vi "Module (Top Level).vi"(8 "error in":errorcluster) -> (0 "error out":errorcluster)   [LabVIEW 2017, in "WinHost.lvlib"]
uses:
  WinHost.lvlib
  User Events/TypeDefs/Shutdown UE FGV Command.ctl
  Global TypeDefs/Registered Modules.ctl
  Public TypeDefs/Messages.ctl
  Public TypeDefs/Module Events.ctl
  <vilib>/NI/STM/SubVIs/MetaDataElement.ctl
  Private TypeDefs/STM Queue Element.ctl
  <vilib>/NI/STM/TCP/TCP Read Options.ctl
  <vilib>/NI/STM/TCP/Write Meta Data (TCP Ref).vi
  <vilib>/NI/STM/TCP/Write Meta Data (TCP Clst).vi
  <vilib>/NI/STM/TCP/Write Message (TCP).vi
  <vilib>/NI/STM/TCP/Read Message (TCP).vi
  Error Handler/Error Handler.lvlib
  Logger/Logger.lvlib
  Controller/Controller.lvlib
  <vilib>/NI/STM/NI STM.lvlib
  mypam/myPAM.lvlib
  Game/Game.lvlib
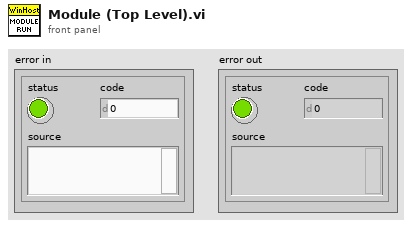
[diagram p1: front panel]
types:
  T1 = typedef "Registered Modules.ctl" = enum16{"Controller", "DAQ", "Error Handler", "Game", "myPAM", "WinHost", "Logger"}
  T2 = typedef "Shutdown UE FGV Command.ctl" = enum16{"create", "get", "destroy"}
  T3 = typedef "Controller.lvlib/Module Reference.ctl" = cluster{"calling module":T1, "module queues":T4, "module notifiers":T5}
  T4 = typedef "Controller.lvlib/Module Queues.ctl" = cluster{"message queue":refnum<queue>}
  T5 = typedef "Controller.lvlib/Module Notifiers.ctl" = cluster{"dummy notifier":refnum<notifier>}
  T6 = typedef "Logger.lvlib/Module Reference.ctl" = cluster{"calling module":T1, "module queues":T7, "module notifiers":T8}
  T7 = typedef "Logger.lvlib/Module Queues.ctl" = cluster{"message queue":refnum<queue>}
  T8 = typedef "Logger.lvlib/Module Notifiers.ctl" = cluster{"dummy notifier":refnum<notifier>}
  T9 = typedef "WinHost.lvlib/Module Reference.ctl" = cluster{"calling module":T1, "module queues":T10, "module notifiers":T11}
  T10 = typedef "WinHost.lvlib/Module Queues.ctl" = cluster{"message queue":refnum<queue>, "STM queue":refnum<queue>}
  T11 = typedef "WinHost.lvlib/Module Notifiers.ctl" = cluster{"dummy notifier":refnum<notifier>}
  T12 = typedef "Error Handler.lvlib/Module Reference.ctl" = cluster{"calling module":T1, "module queues":T13, "module notifiers":T14}
  T13 = typedef "Error Handler.lvlib/Module Queues.ctl" = cluster{"message queue":refnum<queue>}
  T14 = typedef "Error Handler.lvlib/Module Notifiers.ctl" = cluster{"dummy notifier":refnum<notifier>}
  T15 = typedef "WinHost.lvlib/Module Events.ctl" = enum16{"host connected", "enable assistance", "disable assistance", "host disconnected"}
  T16 = typedef "WinHost.lvlib/STM Queue Element.ctl" = cluster{"name":string, "data":string, "stop":bool}
  T17 = typedef "NI STM.lvlib/TCP Read Options.ctl" = cluster{"ignore timeout error":bool, "timeout ms (1000)":i32}
  T18 = typedef "WinHost.lvlib/Messages.ctl" = enum16{"shutdown", "wait for host", "communicate"}
  T19 = typedef "NI STM.lvlib/MetaDataElement.ctl" = string
  T20 = typedef "NI STM.lvlib/TCP Connection Info.ctl" = cluster{"connection ID":refnum<k5>, "meta data":T19[]}
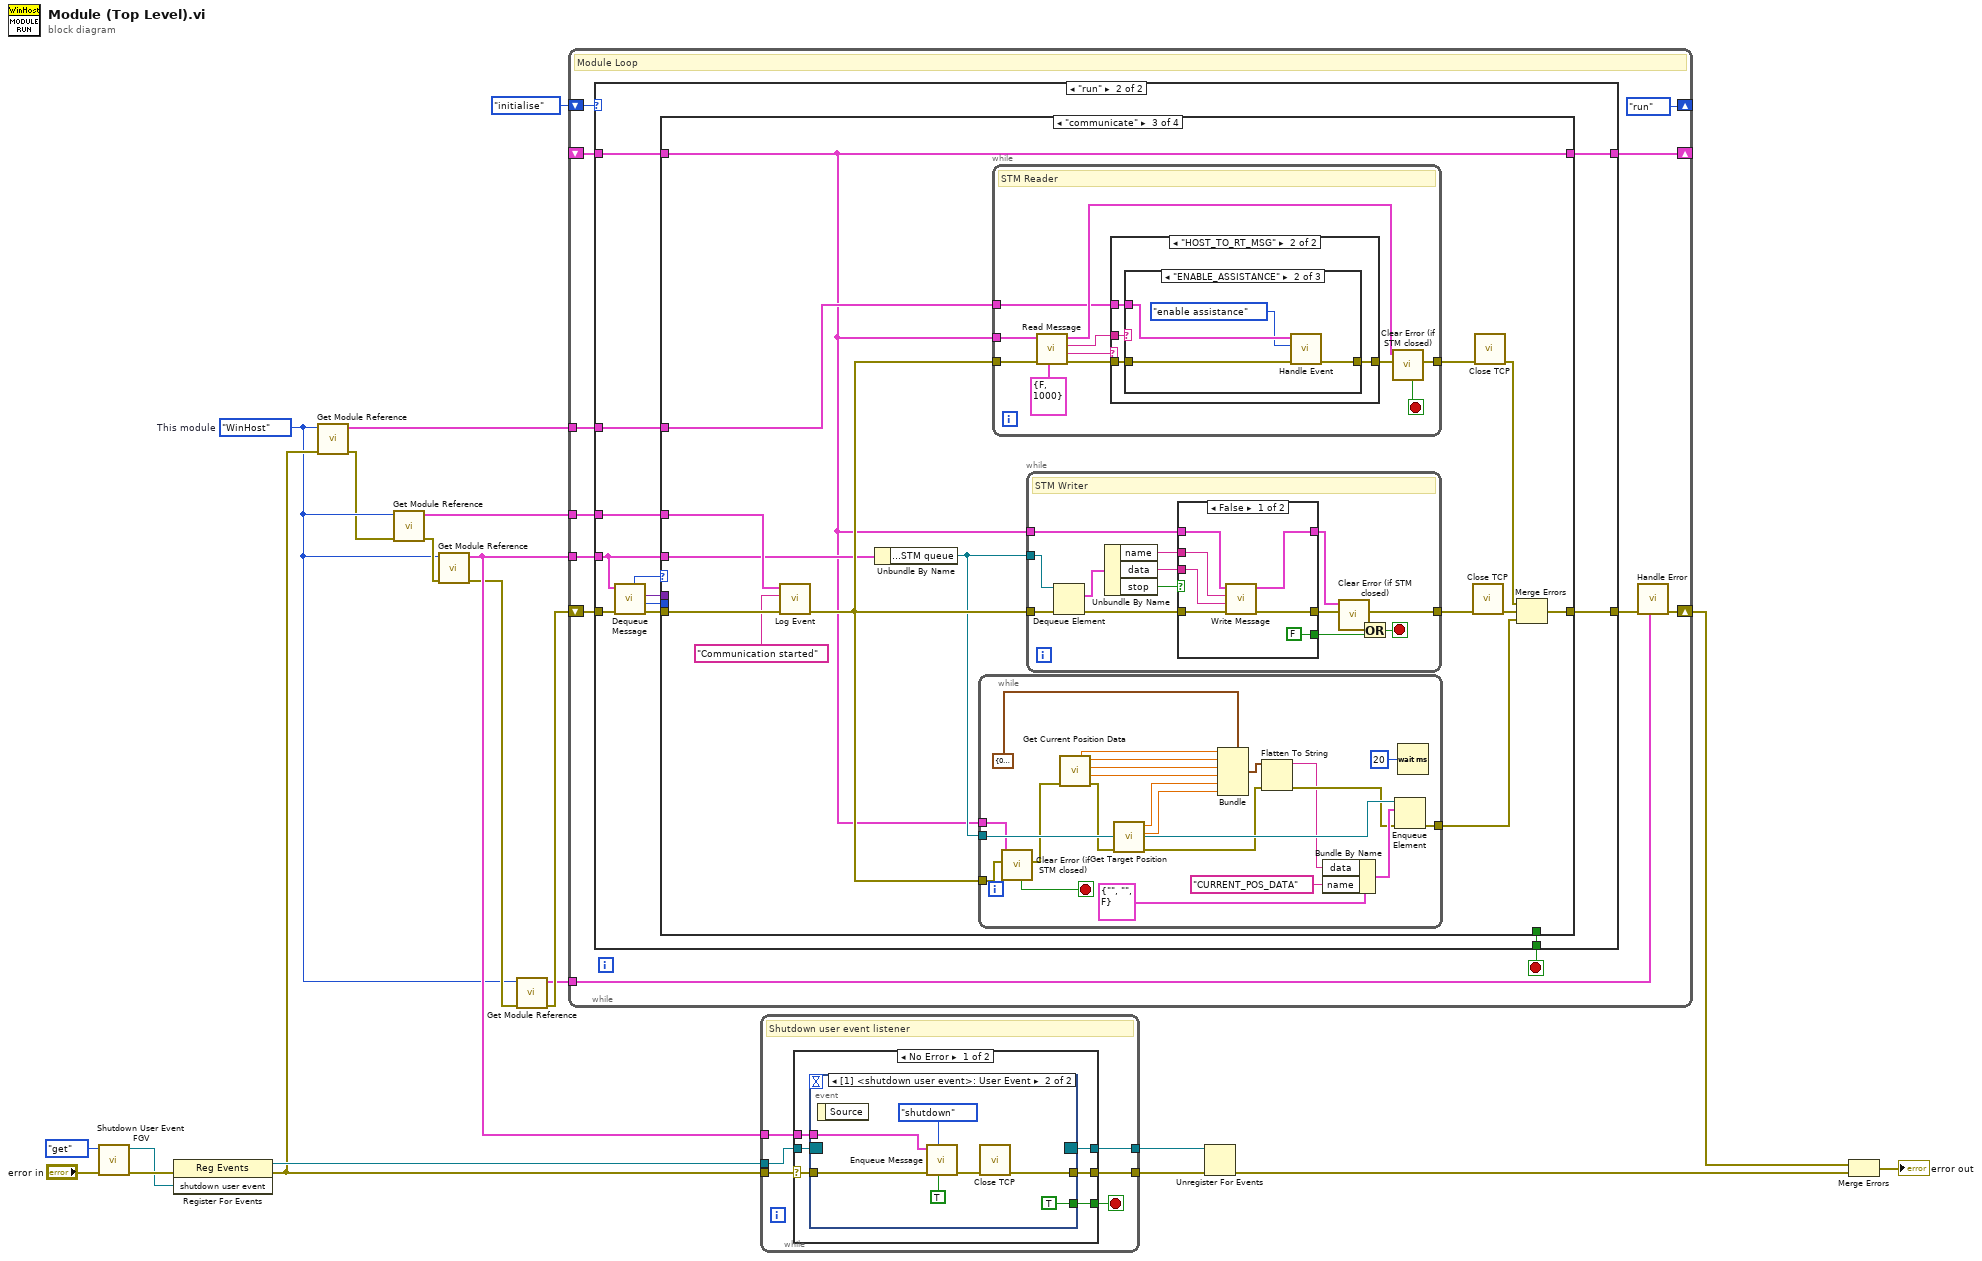
[diagram p0: block diagram]
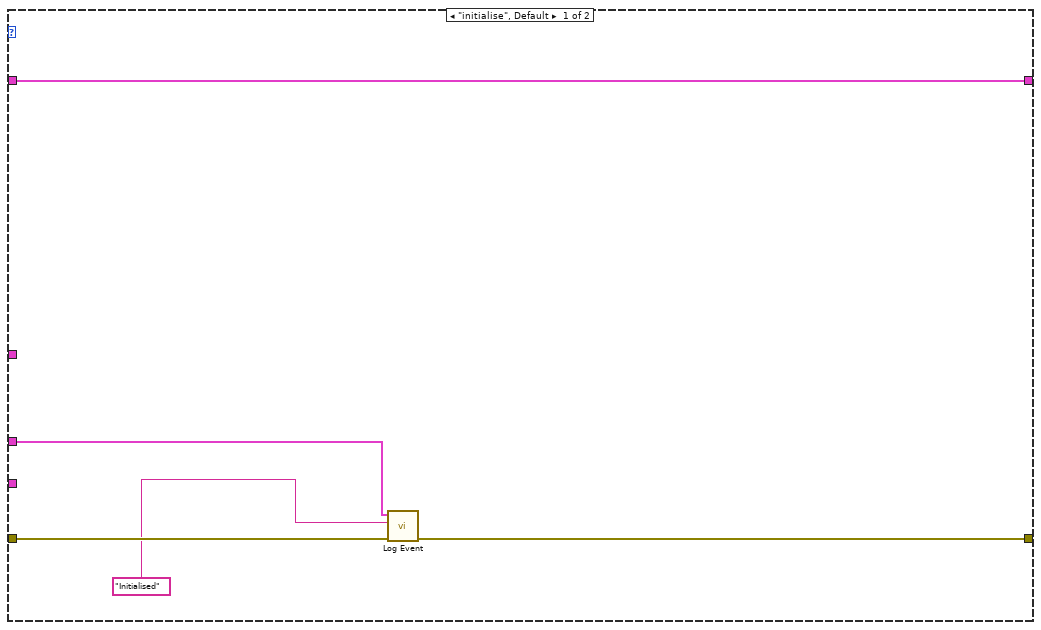
[diagram p2: hidden frame]
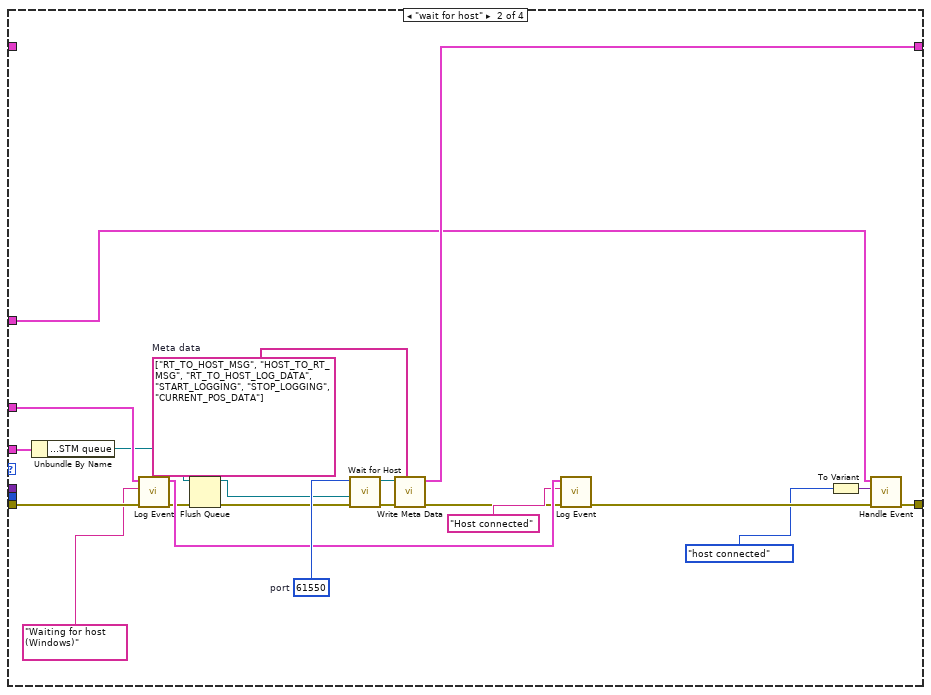
[diagram p4: hidden frame]
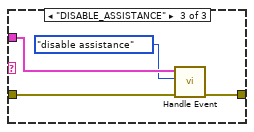
[diagram p7: hidden frame]
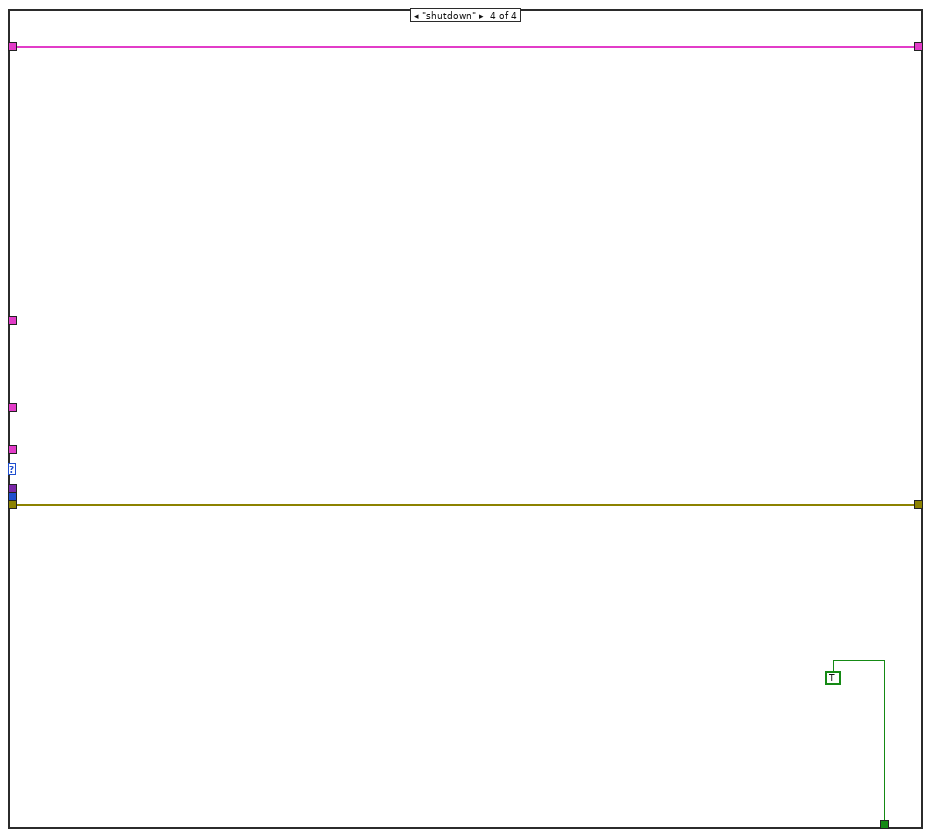
[diagram p9: hidden frame]
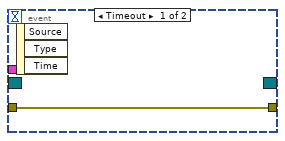
[diagram p10: hidden frame]
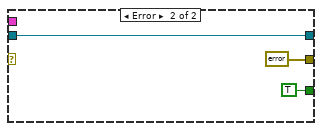
[diagram p11: hidden frame]
diagram:
  w3 = Registered_Modules."WinHost"  # This module
  n1 = call "Shutdown User Event FGV.vi"("error in"="error in", "command"=Shutdown_UE_FGV_Command."get" ("Command")) -> ("error out"=w17:errorcluster, "shutdown user event"=w16:refnum<user-event>)  [unwired: 8 in]
  n2 = register-events(error in=w17, w16) -> (reference out=w20:refnum<event-registration>, error out=w4:errorcluster)  [unwired: 1 in]
  n3 = call "Get Module Reference.vi"("error in"=w4, "calling module"=w3) -> ("error out"=w2:errorcluster, "module reference"=w1:T3)  [unwired: 8 in]
  n4 = call "Get Module Reference.vi"("error in"=w2, "calling module"=w3) -> ("error out"=w9:errorcluster, "module reference"=w11:T6)  [unwired: 8 in]
  n5 = call "Get Module Reference.vi"("error in"=w9, "calling module"=w3) -> ("error out"=w7:errorcluster, "module reference"=w12:T9)  [unwired: 8 in]
  n6 = call "Get Module Reference.vi"("error in"=w7, "calling module"=w3) -> ("error out"=w6:errorcluster, "module reference"=w5:T12)  [unwired: 8 in]
  n7 = while {
    shift-right: [w29] -> w10
    shift-left: w6 -> [w27]
    tunnel: w12 -> [w33]
    tunnel: w11 -> [w32]
    shift-right: [enum16{"initialise", "run"}."run"] -> _
    shift-left: enum16{"initialise", "run"}."initialise" -> [w31]
    tunnel: w5 -> [w25]
    shift-right: [w24] -> _
    shift-left: _ -> [w23]
    tunnel: w1 -> [w22]
    stop <- w26 stop-if-true
    # "Module Loop"
    n8 = case shown="\"run\"" w31 {
      tunnel: [w37 w50] -> w30
      tunnel: w33 -> [_ w40]
      tunnel: w32 -> [w36 w45]
      tunnel: w27 -> [w38 w44]
      tunnel: [_ w43] -> w26
      tunnel: [w34 w42] -> w24
      tunnel: w23 -> [w34 w41]
      tunnel: w22 -> [_ w39]
      frame "initialise", Default {
        n9 = call "Log Event.vi"("error in"=w38, "event"="Initialised", "module reference in"=w36) -> ("error out"=w37:errorcluster)  [unwired: 7 in, 1 out]
      }
      frame "run" {
        n10 = call "Dequeue Message.vi"("error in"=w44, "module reference in"=w40) -> ("error out"=w48:errorcluster, "source"=w46:T1, "data"=w47:variant, "message"=w49:T18)  [unwired: 5 in, 1 out]
        n11 = case shown="\"communicate\"" w49 {
          tunnel: [w52 w66 w84 w161] -> w50
          tunnel: w48 -> [w52 w73 w82 w161]
          tunnel: w47 -> [_ _ _ _]
          tunnel: w46 -> [_ _ _ _]
          tunnel: w45 -> [_ w72 w81 _]
          tunnel: [_ _ _ TRUE] -> w43
          tunnel: [w51 w59 w74 w159] -> w42
          tunnel: w41 -> [w51 _ w74 w159]
          tunnel: w40 -> [_ w58 w75 _]
          tunnel: w39 -> [_ w54 w79 _]
          frame Default {
          }
          frame "wait for host" {
            w63 = T19[] ["RT_TO_HOST_MSG", "HOST_TO_RT_MSG", "RT_TO_HOST_LOG_DATA", "START_LOGGING", "STOP_LOGGING", "CURRENT_POS_DATA"]  # Meta data
            w70 = u16 61550  # port
            n12 = Unbundle By Name(w58) -> ("module queues.STM queue"=w55:refnum<queue>)
            n13 = call "Log Event.vi"("error in"=w73, "event"="Waiting for host (Windows)", "module reference in"=w72) -> ("error out"=w56:errorcluster, "module reference out"=w69:T6)  [unwired: 7 in]
            n14 = Flush Queue(queue=w55, error in (no error)=w56) -> (queue out=w53:refnum<queue>, error out=w57:errorcluster)  [unwired: 1 out]
            n15 = call "Wait for Host.vi"("error in"=w57, "STM queue"=w53, "local tcp port"=w70) -> ("error out"=w62:errorcluster, "connection ID"=w61:refnum<k5>)  [unwired: 7 in]
            n16 = call-poly <vilib>:"Write Meta Data.vi"("meta data"=w63, "error in"=w62, "connection ID"=w61) -> ("error out"=w60:errorcluster, "connection info out"=w59:T20)  [unwired: 2 in, 5 out]
            n17 = call "Log Event.vi"("error in"=w60, "event"="Host connected", "module reference in"=w69) -> ("error out"=w67:errorcluster)  [unwired: 7 in, 1 out]
            n18 = To Variant(anything=Module_Events."host connected" ("module events")) -> (Variant=w65:variant)
            n19 = call "Handle Event.vi"("error in"=w67, "event"=w65, "module reference in"=w54) -> ("error out"=w66:errorcluster)  [unwired: 7 in, 1 out]
          }
          frame "communicate" {
            n20 = call "Log Event.vi"("error in"=w82, "event"="Communication started", "module reference in"=w81) -> ("error out"=w78:errorcluster)  [unwired: 7 in, 1 out]
            n21 = Unbundle By Name(w75) -> ("module queues.STM queue"=w77:refnum<queue>)
            n22 = while {
              tunnel: w78 -> [w96]
              tunnel: w77 -> [w109]
              tunnel: [w107] -> w76
              tunnel: w74 -> [w97]
              stop <- w89 stop-if-true
              n23 = call "Clear Error (if STM closed).vi"("error in"=w96, "stm connection"=w97) -> ("error out"=w95:errorcluster, "stop?"=w89:bool)  [unwired: 8 in]
              n24 = call "Get Current Position Data.vi"("error in"=w95) -> ("link 1 x (mm)"=w106:dbl, "link 1 y (mm)"=w88:dbl, "link 2 x (mm)"=w105:dbl, "link 2 y (mm)"=w104:dbl, "error out"=w94:errorcluster)  [unwired: 10 in]
              n25 = call "Get Target Position.vi"("error in"=w94) -> ("error out"=w93:errorcluster, "target y (mm)"=w90:dbl, "target x (mm)"=w91:dbl)  [unwired: 8 in]
              n26 = Bundle(cluster=cluster{dbl, dbl, dbl, dbl, dbl, dbl} {0.0, 0.0, 0.0, 0.0, 0.0, 0.0}, w106, w88, w105, w104, w91, w90) -> (w101:cluster{dbl, dbl, dbl, dbl, dbl, dbl})
              n27 = Flatten To String(anything=w101, error in (no error)=w93) -> (data string=w99:string, error out=w100:errorcluster)  [unwired: 2 in, 1 out]
              n28 = Bundle By Name(cluster=T16 {"name"="", "data"="", "stop"=FALSE} ("element"), "data"=w99, "name"="CURRENT_POS_DATA") -> (w102:T16)
              n29 = Enqueue Element(queue=w109, element=w102, error in (no error)=w100) -> (error out=w107:errorcluster)  [unwired: 1 in, 2 out]
              n30 = Wait (ms)(milliseconds to wait=u32 20) -> ()  [unwired: 1 out]
            }
            n31 = while {
              tunnel: w74 -> [w120]
              tunnel: w78 -> [w118]
              tunnel: [w113] -> w86
              tunnel: w79 -> [w111]
              stop <- w114 stop-if-true
              # "STM Reader"
              n32 = call-poly <vilib>:"Read Message.vi"("options"=T17 {"ignore timeout error"=FALSE, "timeout ms (1000)"=1000}, "error in"=w118, "connection info in"=w120) -> ("error out"=w116:errorcluster, "name"=w110:T19, "data string"=w117:string, "connection info out"=w112:T20)  [unwired: 3 in, 2 out]
              n33 = case shown="\"HOST_TO_RT_MSG\"" w110 {
                tunnel: w117 -> [_ w125]
                tunnel: w116 -> [w121 w124]
                tunnel: [w121 w123] -> w115
                tunnel: w111 -> [_ w122]
                frame Default {
                }
                frame "HOST_TO_RT_MSG" {
                  n34 = case shown="\"ENABLE_ASSISTANCE\"" w125 {
                    tunnel: w124 -> [w126 w129 w133]
                    tunnel: [w126 w128 w132] -> w123
                    tunnel: w122 -> [_ w130 w134]
                    frame Default {
                      # "Do something with data"
                    }
                    frame "ENABLE_ASSISTANCE" {
                      n35 = call "Handle Event.vi"("error in"=w129, "event"=Module_Events."enable assistance" ("module events"), "module reference in"=w130) -> ("error out"=w128:errorcluster)  [unwired: 7 in, 1 out]
                    }
                    frame "DISABLE_ASSISTANCE" {
                      n36 = call "Handle Event.vi"("error in"=w133, "event"=Module_Events."disable assistance" ("module events"), "module reference in"=w134) -> ("error out"=w132:errorcluster)  [unwired: 7 in, 1 out]
                    }
                  }
                }
              }
              n37 = call "Clear Error (if STM closed).vi"("error in"=w115, "stm connection"=w112) -> ("error out"=w113:errorcluster, "stop?"=w114:bool)  [unwired: 8 in]
            }
            n38 = while {
              tunnel: w77 -> [w147]
              tunnel: w78 -> [w148]
              tunnel: w74 -> [w141]
              tunnel: [w139] -> w87
              stop <- w135 stop-if-true
              # "STM Writer"
              n39 = Dequeue Element(queue=w147, error in (no error)=w148) -> (element=w145:T16, error out=w146:errorcluster)  [unwired: 1 in, 2 out]
              n40 = Unbundle By Name(w145) -> ("name"=w143:string, "data"=w142:string, "stop"=w144:bool)
              n41 = case shown="False" w144 {
                selector: w144 -> [_ w157]
                tunnel: w146 -> [w155 w158]
                tunnel: w143 -> [w153 _]
                tunnel: w142 -> [w152 _]
                tunnel: [w154 w158] -> w140
                tunnel: [FALSE w157] -> w138
                tunnel: w141 -> [w150 w156]
                tunnel: [w149 w156] -> w137
                frame False {
                  n42 = call-poly <vilib>:"Write Message.vi"("error in"=w155, "data"=w152, "name"=w153, "connection info in"=w150) -> ("error out"=w154:errorcluster, "connection info out"=w149:T20)  [unwired: 6 in]
                }
                frame True {
                }
              }
              n43 = call "Clear Error (if STM closed).vi"("error in"=w140, "stm connection"=w137) -> ("error out"=w139:errorcluster, "stop?"=w136:bool)  [unwired: 8 in]
              n44 = Or(x=w136, y=w138) -> (x .or. y?=w135:bool)
            }
            n45 = call "Close TCP.vi"("error in"=w87) -> ("error out"=w85:errorcluster)  [unwired: 10 in]
            n46 = call "Close TCP.vi"("error in"=w86) -> ("error out"=w83:errorcluster)  [unwired: 10 in]
            n47 = Merge Errors(w83, w85, w76) -> (w84:errorcluster)
          }
          frame "shutdown" {
          }
        }
      }
    }
    n48 = call "Handle Error.vi"("module reference in"=w25, "error in"=w30) -> ("error out"=w29:errorcluster)  [unwired: 9 in]
  }
  n49 = while {
    tunnel: w20 -> [w167]
    tunnel: [w166] -> w19
    tunnel: w4 -> [w164]
    tunnel: [w163] -> w14
    tunnel: w12 -> [w162]
    stop <- w165 stop-if-true
    # "Shutdown user event listener"
    n50 = case shown="No Error" w164 {
      selector: w164 -> [w170 _]
      tunnel: w167 -> [w173 w183]
      tunnel: [w172 w183] -> w166
      tunnel: [w171 TRUE] -> w165
      tunnel: [w169 errorcluster {"status"=FALSE, "code"=0, "source"=""} ("error out")] -> w163
      tunnel: w162 -> [w168 _]
      frame No Error {
        n51 = event shown="[1] <shutdown user event>: User Event" {
          selector: w173 -> [_ _]
          dyn-events: [_ _] -> w172
          timeout: _ -> [_ _]
          tunnel: w170 -> [w174 w179]
          tunnel: [w174 w175] -> w169
          tunnel: [_ TRUE] -> w171
          tunnel: w168 -> [_ w178]
          event Timeout {
            n52 = event-data() -> ()  [unwired: 1 in, 3 out]
          }
          event User Event {
            n53 = event-data() -> ()  [unwired: 1 in, 1 out]
            n54 = call "Enqueue Message.vi"("high priority"=TRUE, "message"=Messages."shutdown", "error in"=w179, "module reference in"=w178) -> ("error out"=w176:errorcluster)  [unwired: 6 in, 1 out]
            n55 = call "Close TCP.vi"("error in"=w176) -> ("error out"=w175:errorcluster)  [unwired: 10 in]
          }
        }
      }
      frame Error {
      }
    }
  }
  n56 = Unregister For Events(event registration refnum=w19, error in=w14) -> (error out=w15:errorcluster)
  n57 = Merge Errors(w10, w15) -> (→"error out":errorcluster)
